vi "load_full_report.vi"(8 "error in (no error)":errorcluster, 11 "report path":path=path "D:/Comics/data/Complete_CLZ_collection.csv") -> (0 "error out":errorcluster, 3 "clz_comics":T1[](array[typedef]) {"Release Date" format="%<%x>T"})   [LabVIEW 2024, in "CLZ_to_ComicVine.lvlib"]
uses:
  CLZ_to_ComicVine.lvlib
  typedefs/CLZ_comic.ctl
  <vilib>/Utility/error.llb/Trim Whitespace One-Sided.vi
  <vilib>/Utility/file.llb/Read Delimited Spreadsheet (string).vi
  <userlib>/_OpenG.lib/string/string.llb/openg_string.lvlib
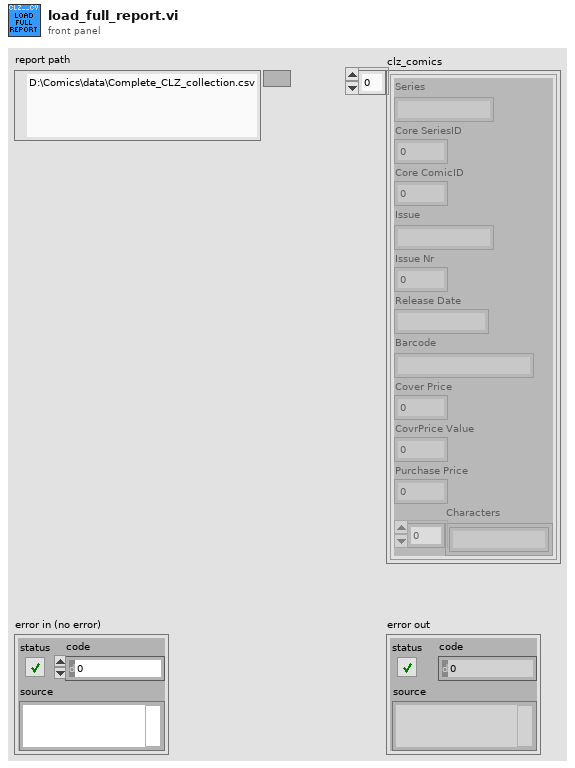
[diagram p1: front panel]
types:
  T1 = typedef "CLZ_to_ComicVine.lvlib/CLZ_comic.ctl" = cluster{"Series":string, "Core SeriesID":i32, "Core ComicID":i32, "Issue":string, "Issue Nr":i32, "Release Date":timestamp, "Barcode":string, "Cover Price":dbl, "CovrPrice Value":dbl, "Purchase Price":dbl, "Characters":string[]}
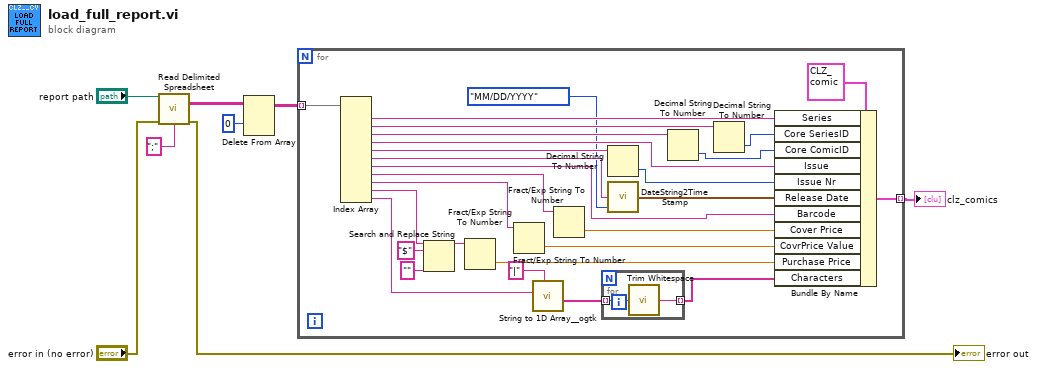
[diagram p0: block diagram]
diagram:
  n1 = call-poly <vilib>:"Read Delimited Spreadsheet.vi"("file path (dialog if empty)"="report path", "error in (no error)"="error in (no error)", "delimiter (\\t)"=";" ("delimiter (\\t)")) -> ("all rows"=w5:string[][], "error out"=→"error out":errorcluster)  [unwired: 7 in, 4 out]
  n2 = Delete From Array(array=w5, index (row)=0) -> (array with subset deleted=w3:string[][])  [unwired: 2 in, 1 out]
  n3 = for {
    tunnel: w3 -> [w36] mode=indexing
    tunnel: [w14] -> w1 mode=indexing
    n4 = Index Array(array=w36) -> (element #1=w34:string, element #2=w33:string, element #3=w31:string, element #4=w29:string, element #5=w28:string, element #6=w26:string, element #7=w24:string, element #8=w23:string, element #9=w21:string, element #10=w12:string, element #11=w18:string)  [unwired: 11 in]
    n5 = Search and Replace String(input string=w12, search string="$", replace string="" ("replace string (\"\")")) -> (result string=w9:string)  [unwired: 5 in, 3 out]
    n6 = Fract/Exp String To Number(string=w9) -> (number=w19:dbl)  [unwired: 3 in, 1 out]
    n7 = Fract/Exp String To Number(string=w21) -> (number=w20:dbl)  [unwired: 3 in, 1 out]
    n8 = call <userlib>:"String to 1D Array__ogtk.vi"("delimiter (Tab)"="|", "string"=w18) -> ("Array of Strings"=w16:string[])  [unwired: 9 in]
    n9 = Fract/Exp String To Number(string=w23) -> (number=w22:dbl)  [unwired: 3 in, 1 out]
    n10 = for {
      tunnel: w16 -> [w38] mode=indexing
      tunnel: [w37] -> w15 mode=indexing
      n11 = call <vilib>:"Trim Whitespace.vi"("string"=w38) -> ("trimmed string"=w37:string)  [unwired: 1 in]
    }
    n12 = Decimal String To Number(string=w28) -> (number=w27:i32)  [unwired: 2 in, 1 out]
    n13 = call "DateString2TimeStamp.vi"("DateFormat"=enum16{"YYYY/MM/DD", "MM/DD/YYYY", "DD/MM/YYYY"}."MM/DD/YYYY", "DateString(YYYY/MM/DD)"=w26) -> ("time stamp"=w25:timestamp)  [unwired: 3 in]
    n14 = Decimal String To Number(string=w31) -> (number=w30:i32)  [unwired: 2 in, 1 out]
    n15 = Decimal String To Number(string=w33) -> (number=w32:i32)  [unwired: 2 in, 1 out]
    n16 = Bundle By Name(cluster=T1 {"Series"="", "Core SeriesID"=0, "Core ComicID"=0, "Issue"="", "Issue Nr"=0, "Release Date"=timestamp(0 s since 1904-01-01), "Barcode"="", "Cover Price"=0.0, "CovrPrice Value"=0.0, "Purchase Price"=0.0, "Characters"=[]} ("CLZ comic"), "Series"=w34, "Core SeriesID"=w32, "Core ComicID"=w30, "Issue"=w29, "Issue Nr"=w27, "Release Date"=w25, "Barcode"=w24, "Cover Price"=w22, "CovrPrice Value"=w20, "Purchase Price"=w19, "Characters"=w15) -> (w14:T1)
  }
  "clz_comics" <- w1
